vi "test_tcp.vi"() -> ()   [LabVIEW 2014]
panel:
  out "initialized array":string[](array[string])
  in  "address":string="localhost"
  in  "Color Box":u32(colorbox)=6618880
  out "data out":string
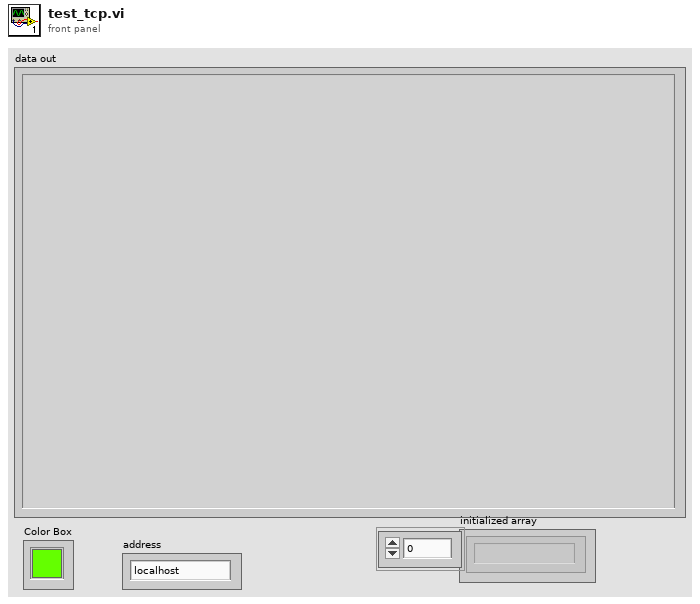
[diagram p1: front panel]
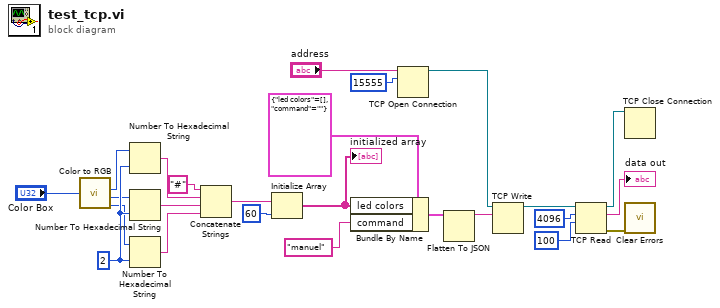
[diagram p0: block diagram]
diagram:
  w10 = i16 2 ("width (-)")
  n1 = call <vilib>:"Color to RGB.vi"("Color"="Color Box") -> ("R"=w11:u8, "G"=w9:u8, "B"=w8:u8)  [unwired: 1 out]
  n2 = Number To Hexadecimal String(1:w10, 2:w11) -> (0:w7:string)
  n3 = Number To Hexadecimal String(1:w10, 2:w9) -> (0:w6:string)
  n4 = Number To Hexadecimal String(1:w10, 2:w8) -> (0:w5:string)
  n5 = Concatenate Strings("#", w7, w6, w5) -> (w3:string)
  n6 = Initialize Array(w3, 60 ("dimension size")) -> (w1:string[])
  "initialized array" <- w1
  n7 = Bundle By Name(cluster=cluster{"led colors":string[], "command":string} {"led colors"=[], "command"=""}, "led colors"=w1, "command"="manuel") -> (w14:cluster{"led colors":string[], "command":string})
  n8 = TCP Open Connection(address="address", remote port or service name=u16 15555) -> (connection ID=w23:refnum<k5>)  [unwired: 3 in, 1 out]
  n9 = Flatten To JSON(anything=w14) -> (JSON string=w22:string)  [unwired: 2 in, 1 out]
  n10 = TCP Write(connection ID=w23, data in=w22) -> (connection ID out=w21:refnum<k5>)  [unwired: 2 in, 2 out]
  n11 = TCP Read(connection ID=w21, bytes to read=4096, 9:100 ("timeout ms (25000)")) -> (connection ID out=w18:refnum<k5>, data out=→"data out":string, error out=w16:errorcluster)  [unwired: 2 in]
  n12 = TCP Close Connection(connection ID=w18) -> ()  [unwired: 2 in, 2 out]
  n13 = call <vilib>:"Clear Errors.vi"("error in (no error)"=w16) -> ()  [unwired: 5 in, 2 out]
